vi "YoutubeCacheProxy.vi"(8 "error in (no error)":errorcluster, 10 "ThirdPartyYoutubeClass.lvclass":refnum<class "ThirdPartyYoutubeClass.lvclass">, 11 "YoutubeCacheProxy in":refnum<class "YoutubeCacheProxy.lvclass">) -> (0 "error out":errorcluster, 3 "YoutubeCacheProxy out":refnum<class "YoutubeCacheProxy.lvclass">)   [LabVIEW 2017, in "YoutubeCacheProxy.lvclass"]
uses:
  YoutubeCacheProxy.lvclass
  ThirdPartyYoutubeClass Class/ThirdPartyYoutubeClass.lvclass
  C:/Users/fflores/Documents/LabVIEW-Open-Projects/LabIVEW OOP Design Patterns/Proxy Pattern/ThirdPartyYoutubeLib Class/ThirdPartyYoutubeLib.lvclass
  YoutubeCacheProxy.lvclass/YoutubeCacheProxy.ctl
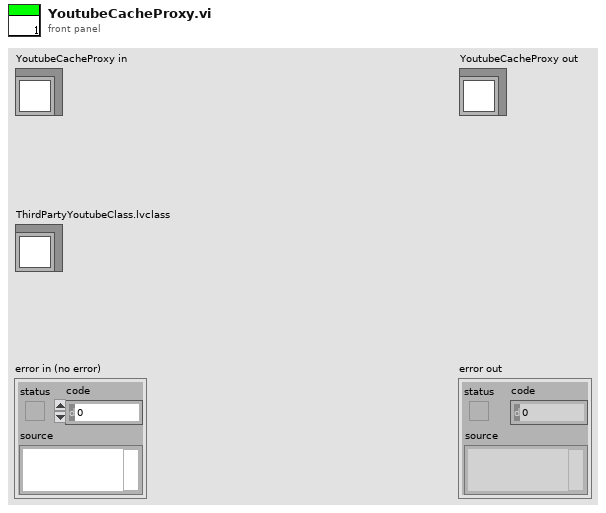
[diagram p1: front panel]
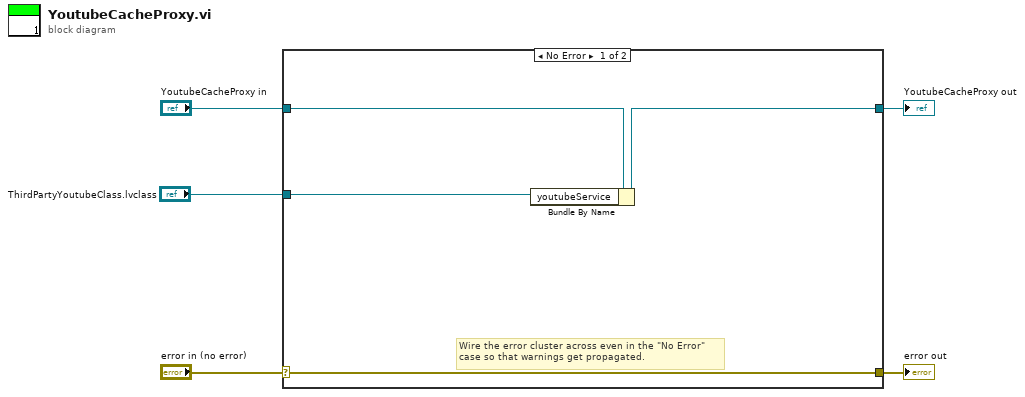
[diagram p0: block diagram]
diagram:
  n1 = case shown="No Error" "error in (no error)" {
    selector: "error in (no error)" -> [w8 w11]
    tunnel: [w8 w11] -> w4
    tunnel: [w7 w10] -> w2
    tunnel: "YoutubeCacheProxy in" -> [w9 w10]
    tunnel: "ThirdPartyYoutubeClass.lvclass" -> [w6 _]
    frame No Error {
      # "Wire the error cluster across even in the \"No Error\"\ncase so that warnings get propagated."
      n2 = Bundle By Name(cluster=w9, "youtubeService"=w6) -> (w7:refnum<class "YoutubeCacheProxy.lvclass">)
    }
    frame Error {
    }
  }
  "error out" <- w4
  "YoutubeCacheProxy out" <- w2
